vi "Write Mission Controller Settings Message.vi"(8 "error in (no error)":errorcluster, 10 "Mission Controller Settings":T1, 11 "Set Mission Controller Settings Message in":refnum<class "Set Mission Controller Settings Message.lvclass">) -> (0 "error out":errorcluster, 3 "Set Mission Controller Settings Message out":refnum<class "Set Mission Controller Settings Message.lvclass">)   [LabVIEW 2015, in "RDS Child Messages.lvlib" / "Set Mission Controller Settings Message.lvclass"]
uses:
  Set Mission Controller Settings Message.lvclass
  RDS Mission Controller Actor/Mission Controller Settings.ctl
  Set Mission Controller Settings Message.lvclass/Set Mission Controller Settings Message.ctl
  RDS Mission Controller Actor/RDS Mission Controller Actor.lvlib
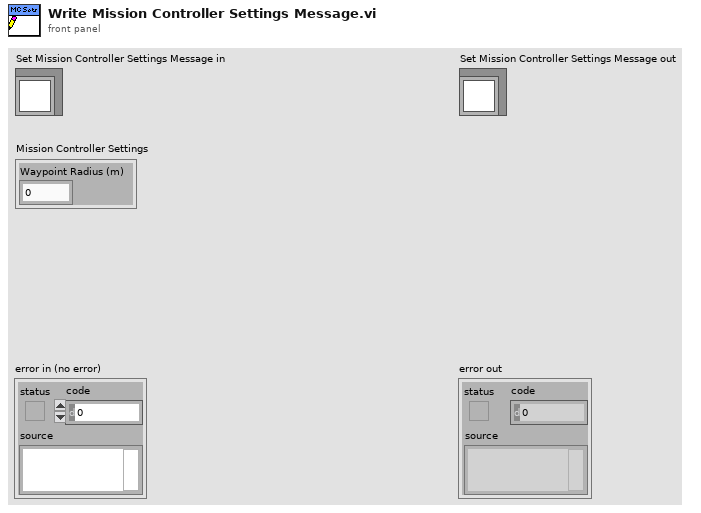
[diagram p1: front panel]
types:
  T1 = typedef "RDS Mission Controller Actor.lvlib/Mission Controller Settings.ctl" = cluster{"Waypoint Radius (m)":dbl}
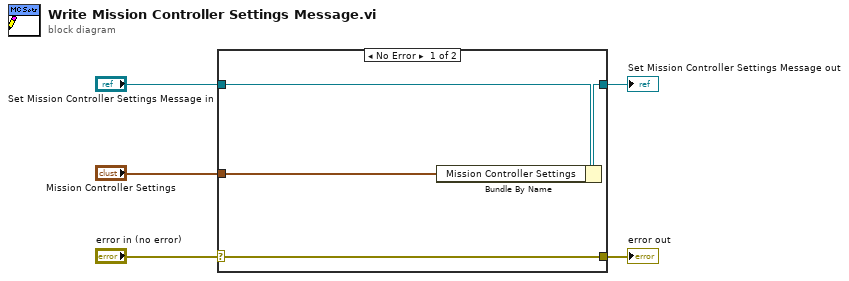
[diagram p0: block diagram]
diagram:
  n1 = case shown="No Error" "error in (no error)" {
    selector: "error in (no error)" -> [w9 w10]
    tunnel: [w9 w10] -> w4
    tunnel: [w7 w11] -> w2
    tunnel: "Set Mission Controller Settings Message in" -> [w8 w11]
    tunnel: "Mission Controller Settings" -> [w6 _]
    frame No Error {
      n2 = Bundle By Name(cluster=w8, "Mission Controller Settings"=w6) -> (w7:refnum<class "Set Mission Controller Settings Message.lvclass">)
    }
    frame Error {
    }
  }
  "error out" <- w4
  "Set Mission Controller Settings Message out" <- w2
